vi "to string.vi"(8 "error in":errorcluster, 11 "configuration in":refnum<class "Template Action Cfg.lvclass">) -> (0 "error out":errorcluster, 1 "data":string, 2 "version":string, 3 "configuration out":refnum<class "Template Action Cfg.lvclass">)   [LabVIEW 2014, in "Template Action Cfg.lvclass"]
doc: "Provides an interface for saving a module configuration to a file or other serialized data source. It is recommended that all children of this class store data in two sets--data required for its own initialization, and any data required for parent initialization--and that each implementation uses the <b>Call Parent Method</b> primitive to serialize parent information."
uses:
  Template Action Cfg.lvclass
  Template Action Cfg.lvclass/Template Action Cfg.ctl
  <vilib>/NI/TBM Modules/Sequencer/sequencer parent classes/action configuration parent/action configuration.lvclass
  <vilib>/NI/Configuration Framework/serializable configuration/NISE_CEF_serializable configuration.lvclass
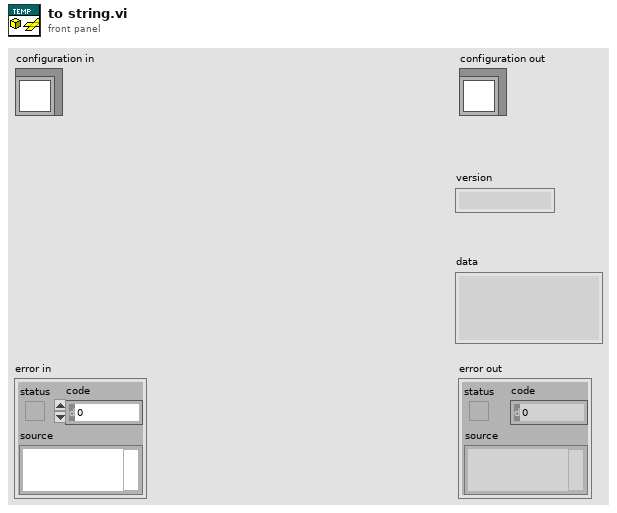
[diagram p1: front panel]
types:
  T1 = typedef "Template Action Cfg.lvclass/configuration data.ctl" = cluster{"Placeholder":dbl}
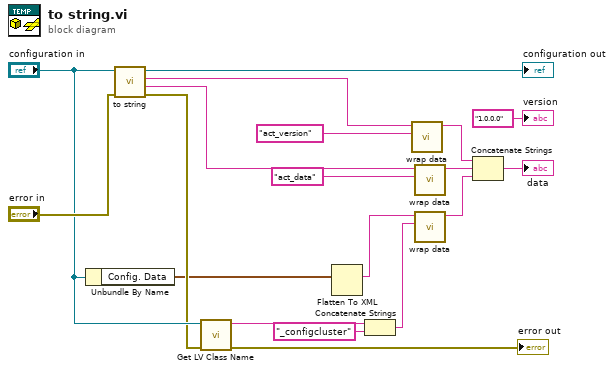
[diagram p0: block diagram]
diagram:
  n1 = Unbundle By Name("configuration in") -> ("Config. Data"=w11:T1)
  n2 = call-parent "to string.vi"("error in"="error in", "configuration in"="configuration in") -> ("error out"=w13:errorcluster, "data"=w6:string, "version"=w9:string, "configuration out"=→"configuration out":refnum<class "Template Action Cfg.lvclass">)  [unwired: 6 in]
  n3 = call <vilib>:"Get LV Class Name.vi"("error in (no error)"=w13, "object"="configuration in") -> ("error out"=→"error out":errorcluster, "class name"=w16:string)  [unwired: 8 in]
  n4 = Flatten To XML(anything=w11) -> (xml string=w3:string)
  n5 = Concatenate Strings(w16, "_configcluster" ("string")) -> (w1:string)
  n6 = call <vilib>:"wrap data.vi"("identifier"="act_version" ("additional identifier"), "data to wrap"=w9) -> ("wrapped data"=w8:string)  [unwired: 9 in]
  n7 = call <vilib>:"wrap data.vi"("identifier"="act_data" ("additional identifier"), "data to wrap"=w6) -> ("wrapped data"=w4:string)  [unwired: 9 in]
  n8 = call <vilib>:"wrap data.vi"("identifier"=w1, "data to wrap"=w3) -> ("wrapped data"=w2:string)  [unwired: 9 in]
  n9 = Concatenate Strings(w8, w4, w2) -> (→"data":string)
  "version" <- "1.0.0.0" ("version")
